vi "IMG_COLOR_FILTER_ARRAY - Type.vi"(8 "error in (no error)":errorcluster, 11 "IMG_COLOR_FILTER_ARRAY":T1) -> (0 "error out":errorcluster, 3 "IMG_COLOR_FILTER_ARRAY_VALUE":i32)   [LabVIEW 2013]
doc: "Description: Returns color filter array type of RAW data.\nType: Integer - Read only.\n\nIMG_COLOR_FILTER_ARRAY.NONE : B/W sensors.\nIMG_COLOR_FILTER_ARRAY.BAYER_RGGB : Regular Bayer RGGB readout.\nIMG_COLOR_FILTER_ARRAY.CMYG : AK Sony sensors.\nIMG_COLOR_FILTER_ARRAY.RGR : 2R+G readout of RGGB sensor.\nIMG_COLOR_FILTER_ARRAY.BAYER_BGGR : Bayer BGGR readout.\nIMG_COLOR_FILTER_ARRAY.BAYER_GRBG : Bayer GRBG readout.\nIMG_COLOR_FILTER_ARRAY.BAYER_GBRG : Bayer GBRG readout."
uses:
  IMG_COLOR_FILTER_ARRAY.ctl
  C:/Projects/Cameras3.x/xiLib/xiLIB_64bit/xiLIB/xiCamLib/API/x64/xiApi.NETX64.dll
  xiLIB_64bit/xiLIB/xiCamLib/API/x64/xiApi.NETX64.dll
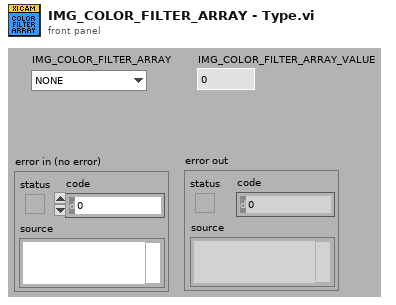
[diagram p1: front panel]
types:
  T1 = typedef "IMG_COLOR_FILTER_ARRAY.ctl" = enum16{"NONE", "BAYER_RGGB", "CMYG", "RGR", "BAYER_BGGR", "BAYER_GRBG", "BAYER_GBRG"}
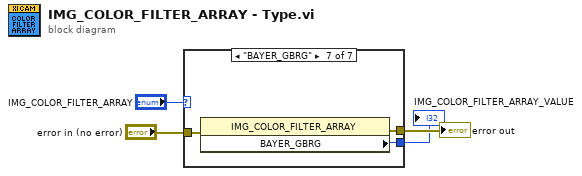
[diagram p0: block diagram]
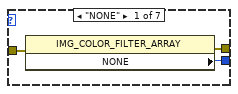
[diagram p2: hidden frame]
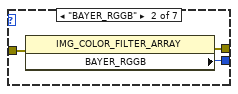
[diagram p3: hidden frame]
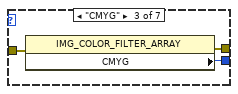
[diagram p4: hidden frame]
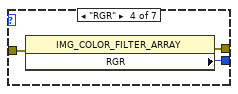
[diagram p5: hidden frame]
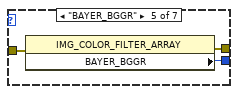
[diagram p6: hidden frame]
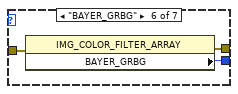
[diagram p7: hidden frame]
diagram:
  n1 = case shown="\"BAYER_GBRG\"" "IMG_COLOR_FILTER_ARRAY" {
    tunnel: "error in (no error)" -> [w7 w10 w13 w16 w19 w22 w25]
    tunnel: [w6 w9 w12 w15 w18 w21 w24] -> w2
    tunnel: [w5 w8 w11 w14 w17 w20 w23] -> w1
    frame "NONE" {
      n2 = property class="IMG_COLOR_FILTER_ARRAY"(error in=w7) -> (error out=w6:errorcluster, "NONE"=w5:i32)  [unwired: 1 in, 1 out]
    }
    frame "BAYER_RGGB" {
      n3 = property class="IMG_COLOR_FILTER_ARRAY"(error in=w10) -> (error out=w9:errorcluster, "BAYER_RGGB"=w8:i32)  [unwired: 1 in, 1 out]
    }
    frame "CMYG" {
      n4 = property class="IMG_COLOR_FILTER_ARRAY"(error in=w13) -> (error out=w12:errorcluster, "CMYG"=w11:i32)  [unwired: 1 in, 1 out]
    }
    frame "RGR" {
      n5 = property class="IMG_COLOR_FILTER_ARRAY"(error in=w16) -> (error out=w15:errorcluster, "RGR"=w14:i32)  [unwired: 1 in, 1 out]
    }
    frame "BAYER_BGGR" {
      n6 = property class="IMG_COLOR_FILTER_ARRAY"(error in=w19) -> (error out=w18:errorcluster, "BAYER_BGGR"=w17:i32)  [unwired: 1 in, 1 out]
    }
    frame "BAYER_GRBG" {
      n7 = property class="IMG_COLOR_FILTER_ARRAY"(error in=w22) -> (error out=w21:errorcluster, "BAYER_GRBG"=w20:i32)  [unwired: 1 in, 1 out]
    }
    frame "BAYER_GBRG" {
      n8 = property class="IMG_COLOR_FILTER_ARRAY"(error in=w25) -> (error out=w24:errorcluster, "BAYER_GBRG"=w23:i32)  [unwired: 1 in, 1 out]
    }
  }
  "error out" <- w2
  "IMG_COLOR_FILTER_ARRAY_VALUE" <- w1
